vi "Set Key Value (RAW).vi"(5 "Key name":string, 6 "Key value":string, 7 "Section name":string, 8 "error in (no error)":errorcluster, 9 "Create key? [T]":bool=TRUE, 10 "Create section? [T]":bool=TRUE, 11 "Carya Config in":refnum<class "Carya Config.lvclass">) -> (0 "error out":errorcluster, 1 "Created key?":bool, 2 "Created session?":bool, 3 "Carya Config out":refnum<class "Carya Config.lvclass">, 4 "Value written?":bool)   [LabVIEW 2013, in "Carya Config.lvclass"]
doc: "Copyright 2018, Carya Automatisering, Wiebe Walstra."
uses:
  Carya Config.lvclass
  Carya Config.lvclass/Carya Config.ctl
  CConfig Object/Loop Query/Loop Query.lvclass
  CConfig Object/CConfig Query.lvclass
  CConfig Object/Insert Query/Insert Query.lvclass
  CConfig Object/Composite Query/Composite Query.lvclass
  CConfig Object/Step In Query/Step In Query.lvclass
  CConfig Object/Set Index Query/Set Index Query.lvclass
  CConfig Object/Set Query/Set Query.lvclass
  CConfig Object/Loop Query/Match Query/Match Query.lvclass
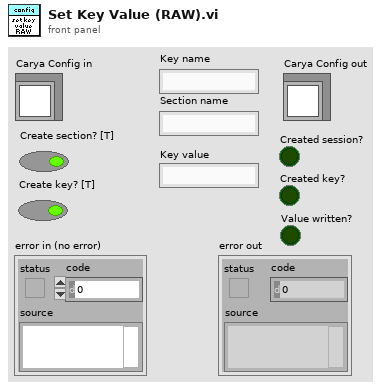
[diagram p1: front panel]
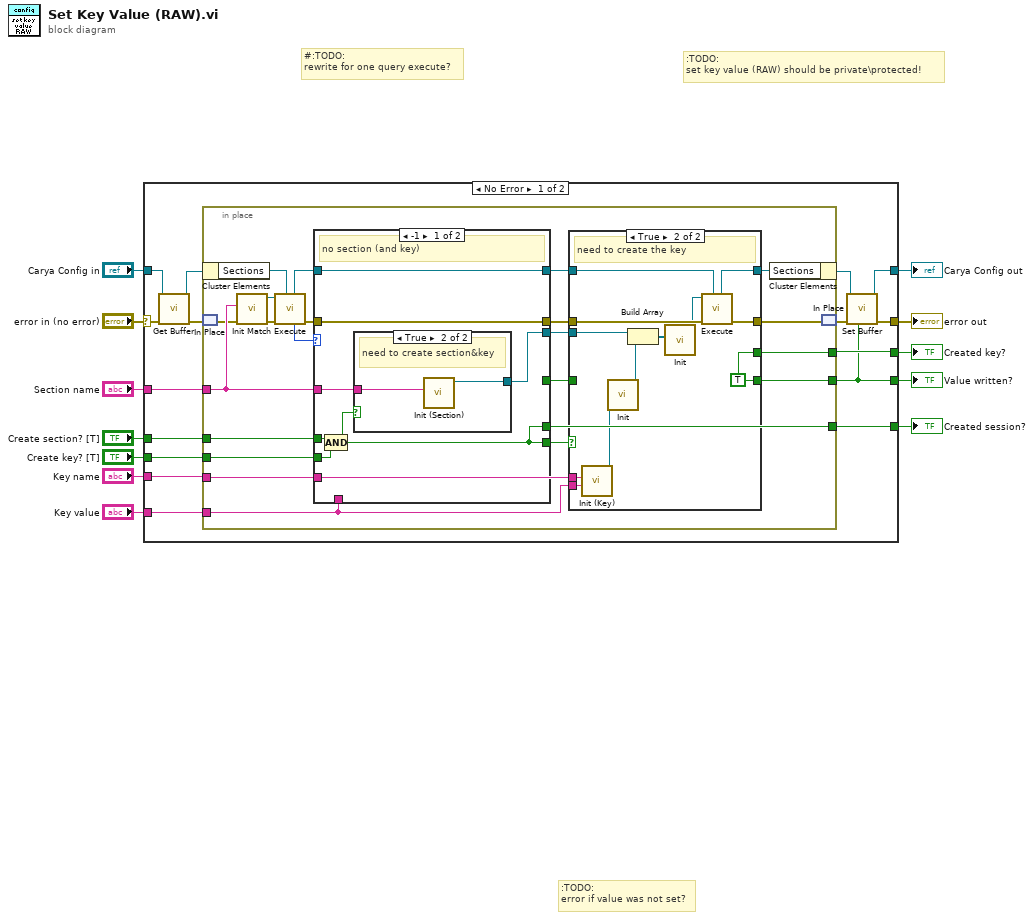
[diagram p0: block diagram]
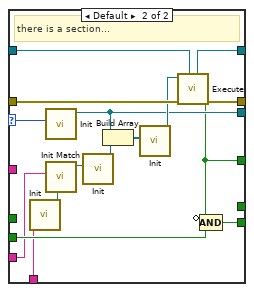
[diagram p4: hidden frame]
diagram:
  # "#:TODO:\nrewrite for one query execute?"
  # ":TODO:\nset key value (RAW) should be private\\protected!"
  # ":TODO:\nerror if value was not set?"
  n1 = case shown="No Error" "error in (no error)" {
    selector: "error in (no error)" -> [w28 w92]
    tunnel: [w19 w92] -> w11
    tunnel: [w18 w91] -> w9
    tunnel: "Carya Config in" -> [w20 w91]
    tunnel: "Section name" -> [w27 _]
    tunnel: "Key name" -> [w26 _]
    tunnel: [w25 _] -> w6
    tunnel: "Key value" -> [w24 _]
    tunnel: "Create key? [T]" -> [w23 _]
    tunnel: "Create section? [T]" -> [w22 _]
    tunnel: [w21 _] -> w2
    tunnel: [w15 _] -> w1
    frame No Error {
      n2 = call-dynamic "Get Buffer.vi"("error in (no error)"=w28, "Carya Config in"=w20) -> ("error out"=w14:errorcluster, "Config"=w16:refnum<class "Carya Config.lvclass">)  [unwired: 8 in]
      n3 = in-place {
        in-place-border: w27 -> [w47]
        in-place-border: w26 -> [w35]
        in-place-border: [w31] -> w25
        in-place-border: w24 -> [w34]
        in-place-border: w23 -> [w45]
        in-place-border: w22 -> [w43]
        in-place-border: [w46] -> w21
        in-place-border: [w30] -> w15
        n4 = in-place-cluster #1(w16) -> ("Sections"=w50:refnum<class "CConfig Object.lvclass">)
        n5 = in-place-match #2(w14) -> (w40:errorcluster)
        n6 = call "Init Match.vi"("error in (no error)"=w40, "Data"=w47) -> ("error out"=w42:errorcluster, "Find First Query out"=w41:refnum<class "Loop Query.lvclass">)  [unwired: 8 in]
        n7 = call-dynamic "Execute.vi"("Composite Object"=w50, "error in (no error)"=w42, "Config Query in"=w41) -> ("error out"=w48:errorcluster, "Index"=w44:i32, "Composite Object"=w49:refnum<class "CConfig Object.lvclass">)  [unwired: 3 in, 3 out]
        n8 = case shown="-1" w44 {
          selector: w44 -> [_ w81]
          tunnel: w49 -> [w67 w87]
          tunnel: [w67 w79] -> w39
          tunnel: [w66 w78] -> w33
          tunnel: w48 -> [w66 w88]
          tunnel: w47 -> [w72 _]
          tunnel: [w68 _] -> w46
          tunnel: w35 -> [_ w82]
          tunnel: w34 -> [_ w83]
          tunnel: w45 -> [w70 w84]
          tunnel: w43 -> [w71 _]
          tunnel: [w69 w77] -> w37
          tunnel: [w68 w76] -> w36
          tunnel: [_ w75] -> w29
          frame -1 {
            # "no section (and key)"
            n9 = Compound Arithmetic op=AND(w71, w70) -> (w68:bool)
            n10 = case shown="True" w68 {
              tunnel: w72 -> [_ w74]
              tunnel: [_ w73] -> w69
              frame False {
                # "done"
              }
              frame True {
                # "need to create section&key"
                n11 = call "Init (Section).vi"("Name"=w74) -> ("Find First Query out"=w73:refnum<class "Insert Query.lvclass">)  [unwired: 9 in, 1 out]
              }
            }
          }
          frame Default {
            # "there is a section..."
            n12 = call "Init.vi"("Value"=w83) -> ("Set Query out"=w85:refnum<class "Set Query.lvclass">)  [unwired: 9 in, 1 out]
            n13 = call "Init.vi"("Index"=w81) -> ("Step In Query out"=w77:refnum<class "Set Index Query.lvclass">)  [unwired: 9 in, 1 out]
            n14 = call "Init Match.vi"("Found"=w85, "Data"=w82) -> ("Find First Query out"=w80:refnum<class "Loop Query.lvclass">)  [unwired: 8 in, 1 out]
            n15 = call "Init.vi"("Config Query"=w80) -> ("Step In Query out"=w90:refnum<class "Step In Query.lvclass">)  [unwired: 9 in, 1 out]
            n16 = Build Array(w77, w90) -> (w89:refnum<class "CConfig Query.lvclass">[])
            n17 = call "Init.vi"("Queries"=w89) -> ("Step In Query out"=w86:refnum<class "CConfig Query.lvclass">)  [unwired: 9 in, 1 out]
            n18 = call-dynamic "Execute.vi"("Composite Object"=w87, "error in (no error)"=w88, "Config Query in"=w86) -> ("error out"=w78:errorcluster, "Result"=w75:bool, "Composite Object"=w79:refnum<class "CConfig Object.lvclass">)  [unwired: 3 in, 3 out]
            n19 = Compound Arithmetic op=AND(invert w75, w84) -> (w76:bool)
          }
        }
        n20 = case shown="True" w36 {
          tunnel: [w51 w58] -> w30
          tunnel: w39 -> [w53 w60]
          tunnel: [w53 w59] -> w38
          tunnel: [w52 w62] -> w32
          tunnel: w33 -> [w52 w63]
          tunnel: [_ w58] -> w31
          tunnel: w37 -> [_ w57]
          tunnel: w35 -> [_ w56]
          tunnel: w34 -> [_ w55]
          tunnel: w29 -> [w51 _]
          frame False {
            # "old key has been written"
          }
          frame True {
            w58 = TRUE ("Result")
            # "need to create the key"
            n21 = call "Init (Key).vi"("Value"=w55, "Name"=w56) -> ("Find First Query out"=w54:refnum<class "Insert Query.lvclass">)  [unwired: 8 in, 1 out]
            n22 = call "Init.vi"("Config Query"=w54) -> ("Step In Query out"=w64:refnum<class "Step In Query.lvclass">)  [unwired: 9 in, 1 out]
            n23 = Build Array(w57, w64) -> (w65:refnum<class "CConfig Query.lvclass">[])
            n24 = call "Init.vi"("Queries"=w65) -> ("Step In Query out"=w61:refnum<class "CConfig Query.lvclass">)  [unwired: 9 in, 1 out]
            n25 = call-dynamic "Execute.vi"("Composite Object"=w60, "error in (no error)"=w63, "Config Query in"=w61) -> ("error out"=w62:errorcluster, "Composite Object"=w59:refnum<class "CConfig Object.lvclass">)  [unwired: 3 in, 4 out]
          }
        }
        n26 = in-place-cluster #1("Sections"=w38) -> (w17:refnum<class "Carya Config.lvclass">)
        n27 = in-place-match #2(w32) -> (w13:errorcluster)
      }
      n28 = call-dynamic "Set Buffer.vi"("Set? [T]"=w15, "error in (no error)"=w13, "Carya Config"=w17) -> ("error out"=w19:errorcluster, "Carya Config out"=w18:refnum<class "Carya Config.lvclass">)  [unwired: 7 in]
    }
    frame Error {
    }
  }
  "error out" <- w11
  "Carya Config out" <- w9
  "Created key?" <- w6
  "Created session?" <- w2
  "Value written?" <- w1
